vi "_CSMObj-Unregister Internal Registry Rules.vi"(5 "CSM:LogFilter.lvclass":refnum<class "LogFilter.lvclass">, 7 "Name (\"\" to Use UUID)":string, 8 "Error In":errorcluster caption="error in (no error)", 10 "CSM Global Log Event":T1, 11 "CSMQ In":T2={"info"={"Module Name"="", "Requested Name"="", "Group Name"="", "Mode"=enum."Stand Alone", "Allowed Messages"=[]}, "Refs"={"WatchDogQ"=refnum, "CSMDataDVR"=refnum, "Queue"={"HPriorityQ"=refnum, "LowPriorityQ"=refnum}, "GroupDataDVR"=refnum, "TagMap"=refnum, "ExitEvent"=refnum, "NewStateEvent"=refnum, "StatusChangeEvent"=refnum}}) -> (0 "error out":errorcluster, 3 "CSMQ Out":T2={"info"={"Module Name"="", "Requested Name"="", "Group Name"="", "Mode"=enum."Stand Alone", "Allowed Messages"=[]}, "Refs"={"WatchDogQ"=refnum, "CSMDataDVR"=refnum, "Queue"={"HPriorityQ"=refnum, "LowPriorityQ"=refnum}, "GroupDataDVR"=refnum, "TagMap"=refnum, "ExitEvent"=refnum, "NewStateEvent"=refnum, "StatusChangeEvent"=refnum}})   [LabVIEW 2017, in "Communicable State Machine.lvlib"]
uses:
  Communicable State Machine.lvlib
  _CSMObj.ctl
  _CSMObj-Info.ctl
  Typedef/_CSM_MODE.ctl
  _CSMObj-Refs.ctl
  _CSMObj-Data.ctl
  Priority Queue/Priority Queue.ctl
  Typedef/_Cross CSM State Data.ctl
  Typedef/_CSM_MSG_TYPE.ctl
  Typedef/_Cross CSM State Response.ctl
  Typedef/_CSM_Response Source Message.ctl
  Priority Queue/def-Data(LowPRI-Q).ctl
  _CSMObj-ModeData.ctl
  Typedef/_CSM Status Change Event Data.ctl
  GlobalEvent/LogFilter/LogFilter.lvclass
  GlobalEvent/GEvt-Refs.ctl
  Typedef/_CSM_GlobalLog_MSG.ctl
  Typedef/_CSM_GlobalLog_MSG_TYPE.ctl
  FGV-BroadcastRegistry/Operation-BroadcastRegistry.ctl
  GlobalEvent/GEvt-Generate with Rule Check.vi
  GlobalEvent/LogFilter/LogFilter - Check.vi
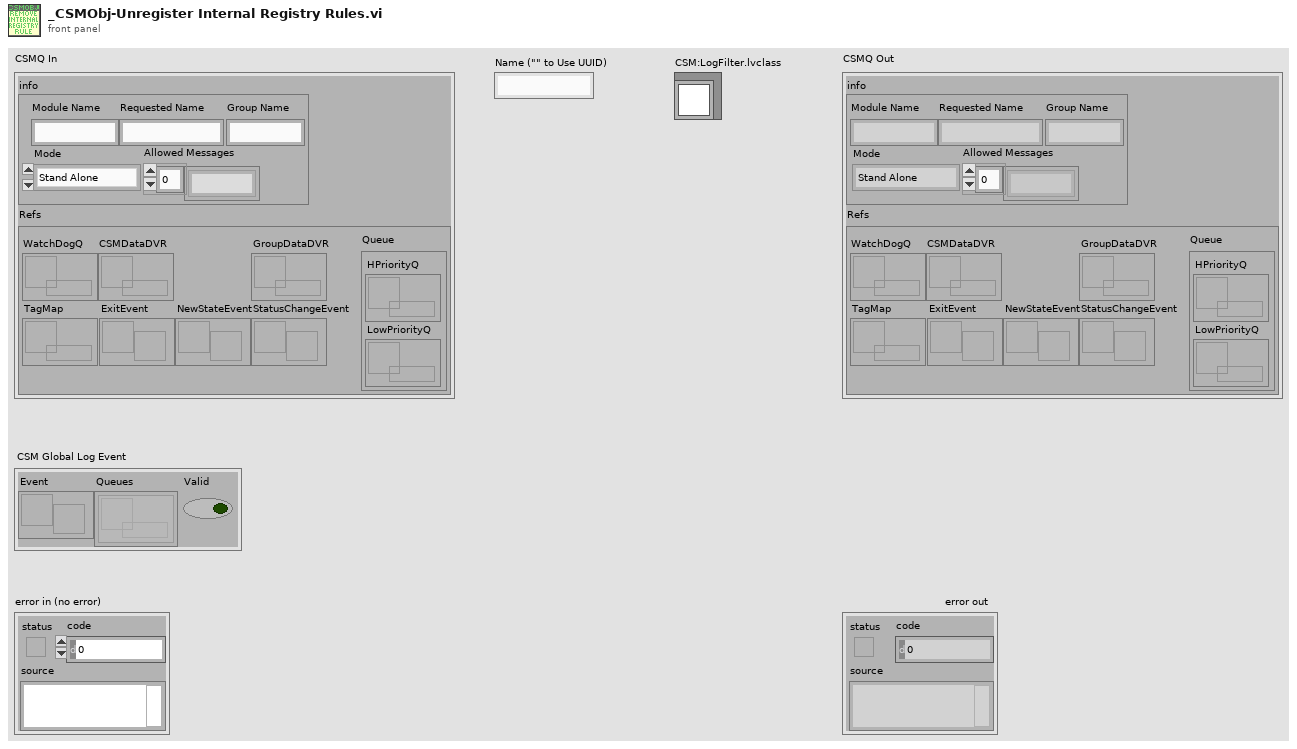
[diagram p1: front panel]
types:
  T1 = typedef "Communicable State Machine.lvlib/GEvt-Refs.ctl" = cluster{"Event":refnum<user-event>, "Queues":refnum<queue>[], "Valid":bool}
  T2 = typedef "Communicable State Machine.lvlib/_CSMObj.ctl" = cluster{"info":T3, "Refs":T5}
  T3 = typedef "Communicable State Machine.lvlib/_CSMObj-Info.ctl" = cluster{"Module Name":string, "Requested Name":string, "Group Name":string, "Mode":T4, "Allowed Messages":string[]}
  T4 = typedef "Communicable State Machine.lvlib/_CSM_MODE.ctl" = enum16{"Not Exist", "Stand Alone", "CSM", "Worker", "Worker Agent", "Chain Node", "Chain"}
  T5 = typedef "Communicable State Machine.lvlib/_CSMObj-Refs.ctl" = cluster{"WatchDogQ":refnum<queue>, "CSMDataDVR":refnum<data-value>, "Queue":T6, "GroupDataDVR":refnum<data-value>, "TagMap":refnum<data-value>, "ExitEvent":refnum<user-event>, "NewStateEvent":refnum<user-event>, "StatusChangeEvent":refnum<user-event>}
  T6 = typedef "Communicable State Machine.lvlib/Priority Queue.ctl" = cluster{"HPriorityQ":refnum<queue>, "LowPriorityQ":refnum<queue>}
  T7 = typedef "Communicable State Machine.lvlib/Operation-BroadcastRegistry.ctl" = enum16{"Delete Source Module", "Delete Target Module", "Remove Module", "Register", "Unregister", "Check", "List Status", "List Entries", "List Status Of Source", "Drop"}
  T8 = typedef "Communicable State Machine.lvlib/_CSMObj-Data.ctl" = cluster{"RemoteMessge?":bool, "error":errorcluster, "Return State":string, "Initialized":enum16{"Initializing", "Ready", "Exiting"}, "InternalRegistryRules":string[]}
  T9 = typedef "Communicable State Machine.lvlib/_CSMObj-ModeData.ctl" = cluster{"CSMDataDVR":refnum<data-value>[], "PriorityQueues":T6[], "Messages of Chain Nodes":cluster{"Module Name":string, "Allowed Messages":string[]}[], "Chain Message Mapping Map":variant, "SharedRegistryRules":string[]}
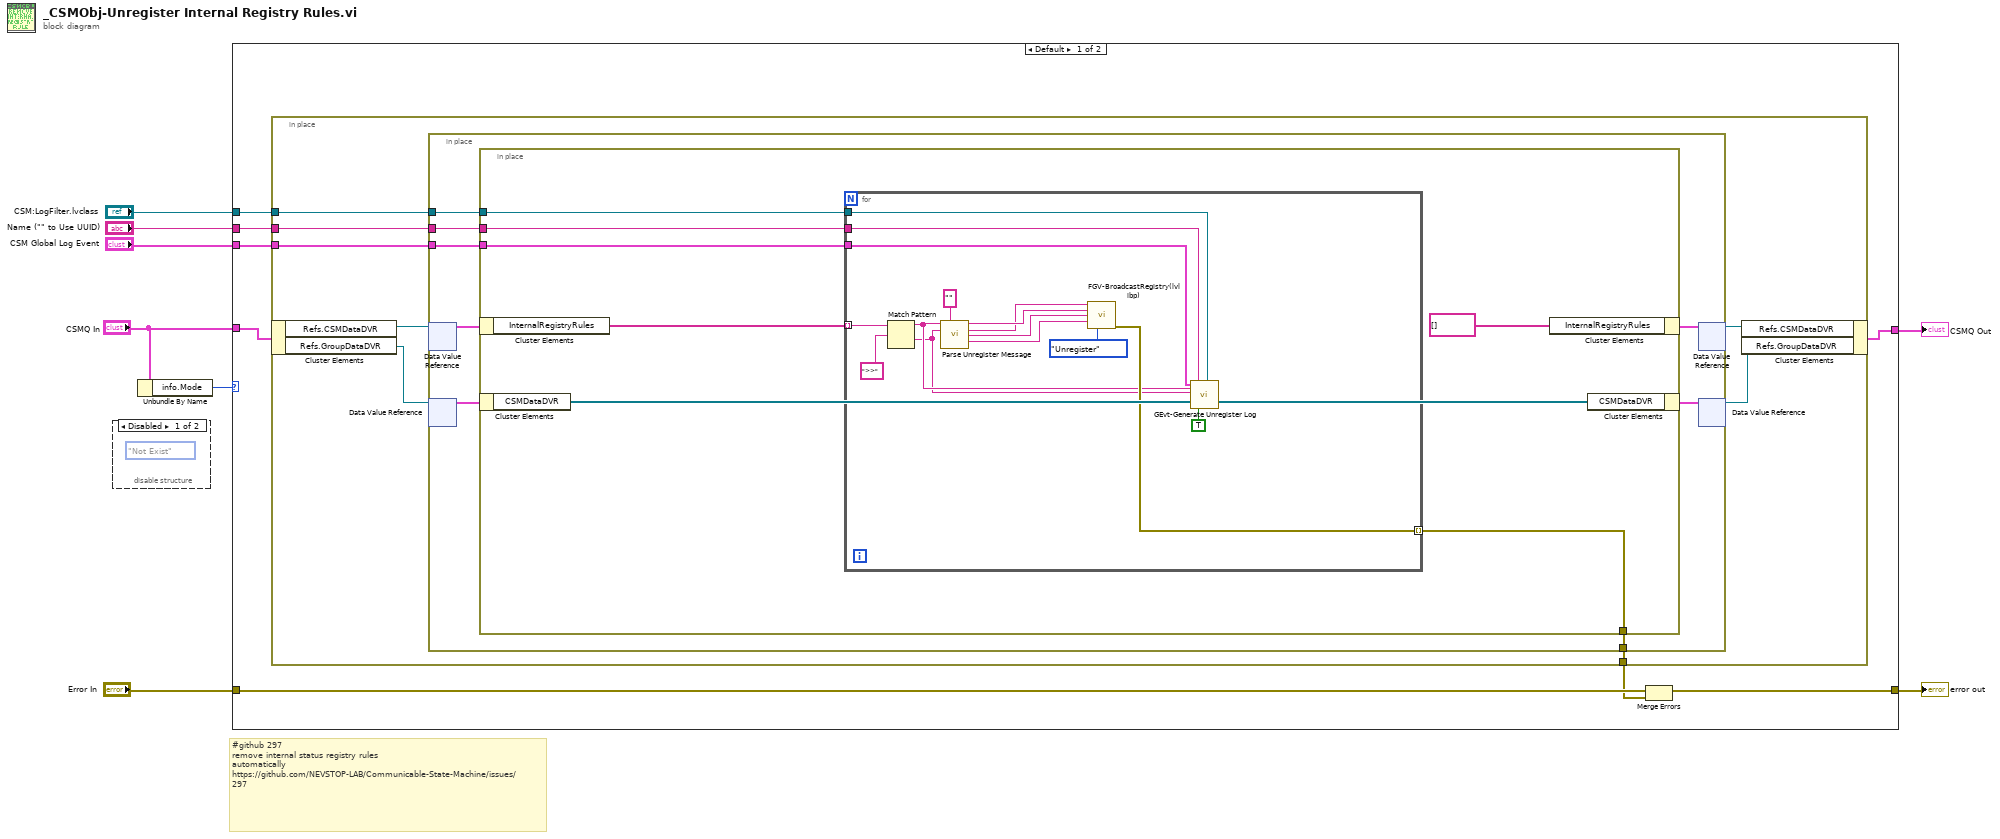
[diagram p0: block diagram]
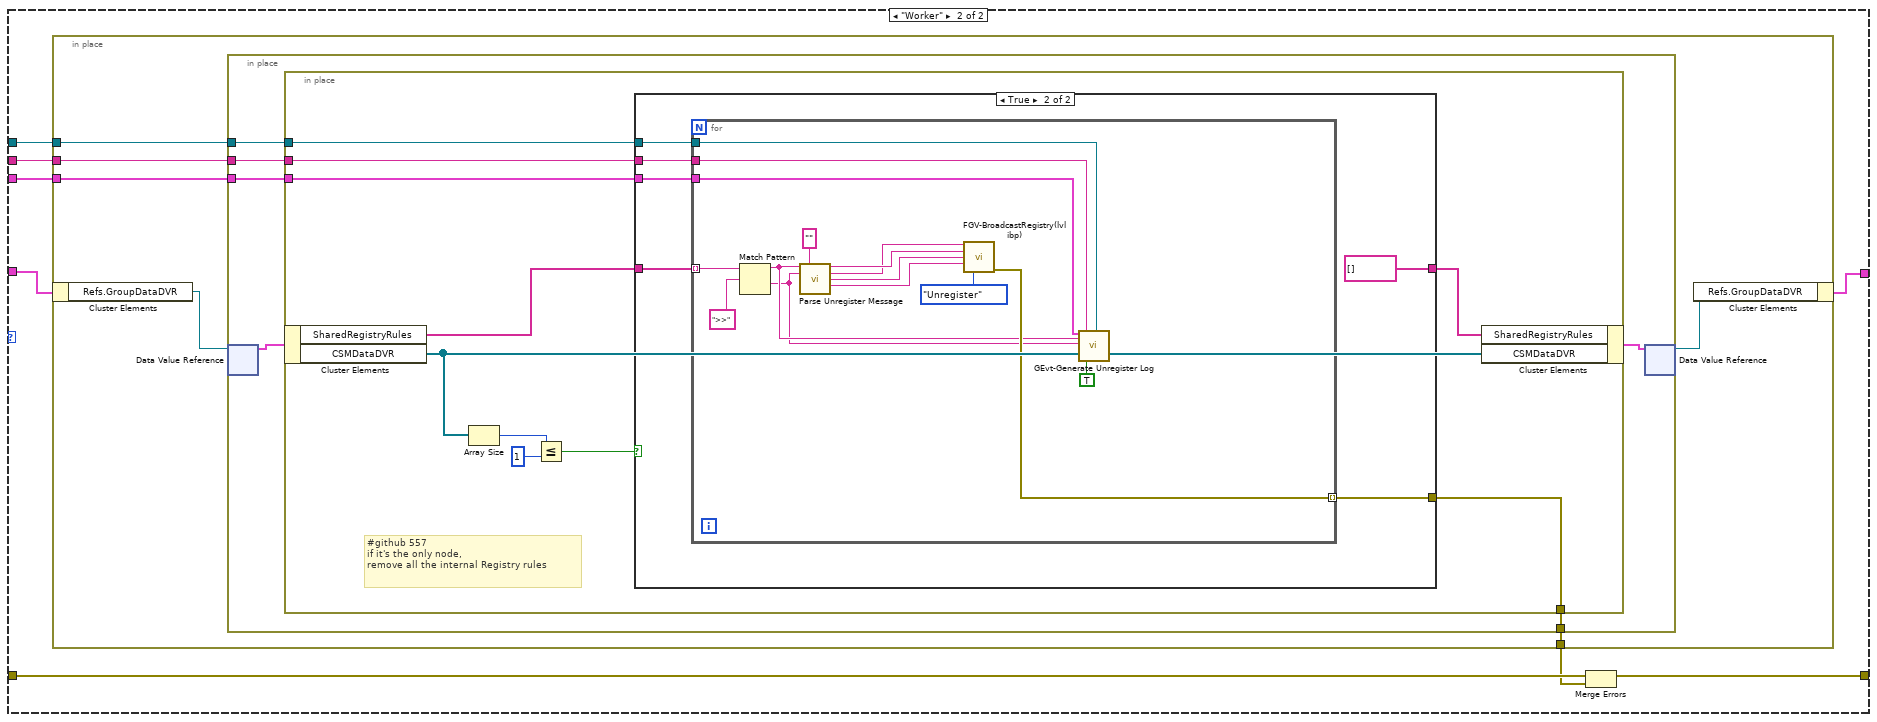
[diagram p3: hidden frame]
diagram:
  # "#github 297\nremove internal status registry rules \nautomatically\nhttps://github.com/NEVSTOP-LAB/Communicable-State-Machine/issues/297"
  n1 = disable-structure shown="Disabled" {
    frame Disabled {
      (unwired) _CSM_MODE."Not Exist" ("Mode")
    }
    frame Enabled {
    }
  }
  n2 = Unbundle By Name("CSMQ In") -> ("info.Mode"=w4:T4)
  n3 = case shown="Default" w4 {
    tunnel: "Error In" -> [w16 w62]
    tunnel: [w15 w61] -> w7
    tunnel: [w14 w60] -> w6
    tunnel: "CSMQ In" -> [w12 w58]
    tunnel: "CSM:LogFilter.lvclass" -> [w11 w57]
    tunnel: "CSM Global Log Event" -> [w10 w56]
    tunnel: "Name (\"\" to Use UUID)" -> [w9 w55]
    frame Default {
      n4 = in-place "In Place Element Structure" {
        in-place-border: [w22] -> w13
        in-place-border: w11 -> [w21]
        in-place-border: w10 -> [w20]
        in-place-border: w9 -> [w19]
        n5 = in-place-cluster #1(w12) -> ("Refs.CSMDataDVR"=w24:refnum<data-value>, "Refs.GroupDataDVR"=w18:refnum<data-value>)
        n6 = in-place {
          in-place-border: [w30] -> w22
          in-place-border: w21 -> [w29]
          in-place-border: w20 -> [w28]
          in-place-border: w19 -> [w27]
          n7 = in-place-dvr #2(w24) -> (w32:T8)  [unwired: 1 out]
          n8 = in-place-dvr #3(w18) -> (w26:T9)  [unwired: 1 out]
          n9 = in-place {
            in-place-border: [w37] -> w30
            in-place-border: w29 -> [w36]
            in-place-border: w28 -> [w35]
            in-place-border: w27 -> [w34]
            n10 = in-place-cluster #4(w32) -> ("InternalRegistryRules"=w38:string[])
            n11 = in-place-cluster #5(w26) -> ("CSMDataDVR"=w33:refnum<data-value>[])
            n12 = for {
              tunnel: w38 -> [w54] mode=indexing
              tunnel: [w46] -> w37 mode=indexing
              tunnel: w36 -> [w45]
              tunnel: w35 -> [w44]
              tunnel: w34 -> [w43]
              n13 = Match Pattern(string=w54, regular expression=">>") -> (before substring=w42:string, after substring=w41:string)  [unwired: 1 in, 2 out]
              n14 = call "Parse Unregister Message.vi"("State"=w42, "Module Name"="", "Args"=w41) -> ("Target"=w51:string, "Source"=w50:string, "Status"=w49:string, "Api"=w48:string)  [unwired: 8 in, 1 out]
              n15 = call "FGV-BroadcastRegistry(lvlibp).vi"("Source"=w50, "Target"=w51, "Status"=w49, "API"=w48, "Operation"=Operation-BroadcastRegistry."Unregister") -> ("error out"=w46:errorcluster)  [unwired: 9 in, 1 out]
              n16 = call "GEvt-Generate Unregister Log.vi"("CSM Global Log Event"=w44, "Current State"=w42, "Arguments"=w41, "Name (\"\" to Use UUID)"=w43, "Remove For Module Exit? (F)"=TRUE ("Remove for Module Exit(F)"), "CSM:LogFilter.lvclass"=w45) -> ()  [unwired: 12 in, 2 out]
            }
            n17 = in-place-cluster #4("InternalRegistryRules"=string[] []) -> (w31:T8)
            n18 = in-place-cluster #5("CSMDataDVR"=w33) -> (w25:T9)
          }
          n19 = in-place-dvr #2(w31) -> (w23:refnum<data-value>)  [unwired: 1 out]
          n20 = in-place-dvr #3(w25) -> (w17:refnum<data-value>)  [unwired: 1 out]
        }
        n21 = in-place-cluster #1("Refs.CSMDataDVR"=w23, "Refs.GroupDataDVR"=w17) -> (w15:T2)
      }
      n22 = Merge Errors(w16, w13) -> (w14:errorcluster)
    }
    frame "Worker" {
      n23 = in-place "In Place Element Structure" {
        in-place-border: [w68] -> w59
        in-place-border: w57 -> [w67]
        in-place-border: w56 -> [w66]
        in-place-border: w55 -> [w65]
        n24 = in-place-cluster #6(w58) -> ("Refs.GroupDataDVR"=w64:refnum<data-value>)
        n25 = in-place {
          in-place-border: [w74] -> w68
          in-place-border: w67 -> [w73]
          in-place-border: w66 -> [w72]
          in-place-border: w65 -> [w71]
          n26 = in-place-dvr #7(w64) -> (w70:T9)  [unwired: 1 out]
          n27 = in-place {
            in-place-border: [w84] -> w74
            in-place-border: w73 -> [w83]
            in-place-border: w72 -> [w82]
            in-place-border: w71 -> [w81]
            # "#github 557\nif it's the only node,\nremove all the internal Registry rules"
            n28 = in-place-cluster #8(w70) -> ("SharedRegistryRules"=w76:string[], "CSMDataDVR"=w77:refnum<data-value>[])
            n29 = Array Size(array=w77) -> (size(s)=w80:i32)
            n30 = Less Or Equal?(x=w80, y=1) -> (x <= y?=w78:bool)
            n31 = case shown="True" w78 {
              tunnel: [w85 string[] [] ("InternalRegistryRules")] -> w75
              tunnel: w76 -> [w85 w90]
              tunnel: [_ w89] -> w84
              tunnel: w83 -> [_ w88]
              tunnel: w82 -> [_ w87]
              tunnel: w81 -> [_ w86]
              frame False {
              }
              frame True {
                n32 = for {
                  tunnel: w90 -> [w106] mode=indexing
                  tunnel: [w98] -> w89 mode=indexing
                  tunnel: w88 -> [w97]
                  tunnel: w87 -> [w96]
                  tunnel: w86 -> [w95]
                  n33 = Match Pattern(string=w106, regular expression=">>") -> (before substring=w94:string, after substring=w93:string)  [unwired: 1 in, 2 out]
                  n34 = call "Parse Unregister Message.vi"("State"=w94, "Module Name"="", "Args"=w93) -> ("Target"=w103:string, "Source"=w102:string, "Status"=w101:string, "Api"=w100:string)  [unwired: 8 in, 1 out]
                  n35 = call "FGV-BroadcastRegistry(lvlibp).vi"("Source"=w102, "Target"=w103, "Status"=w101, "API"=w100, "Operation"=Operation-BroadcastRegistry."Unregister") -> ("error out"=w98:errorcluster)  [unwired: 9 in, 1 out]
                  n36 = call "GEvt-Generate Unregister Log.vi"("CSM Global Log Event"=w96, "Current State"=w94, "Arguments"=w93, "Name (\"\" to Use UUID)"=w95, "Remove For Module Exit? (F)"=TRUE ("Remove for Module Exit(F)"), "CSM:LogFilter.lvclass"=w97) -> ()  [unwired: 12 in, 2 out]
                }
              }
            }
            n37 = in-place-cluster #8("SharedRegistryRules"=w75, "CSMDataDVR"=w77) -> (w69:T9)
          }
          n38 = in-place-dvr #7(w69) -> (w63:refnum<data-value>)  [unwired: 1 out]
        }
        n39 = in-place-cluster #6("Refs.GroupDataDVR"=w63) -> (w61:T2)
      }
      n40 = Merge Errors(w62, w59) -> (w60:errorcluster)
    }
  }
  "error out" <- w6
  "CSMQ Out" <- w7
